vi "Read Item Tag.vi"(8 "error in (no error)":errorcluster, 11 "MenuSelectionMsg in":refnum<class "MenuSelectionMsg.lvclass">) -> (0 "error out":errorcluster, 2 "Item Tag":string, 3 "MenuSelectionMsg out":refnum<class "MenuSelectionMsg.lvclass">)   [LabVIEW 2017, in "ActorEvents.lvlib" / "MenuSelectionMsg.lvclass"]
uses:
  <vilib>/gpm_packages/@cs/mva-viewable/Source/ActorEvents/IEventAggregator Messages/MenuSelectionMsg/MenuSelectionMsg.lvclass
  <vilib>/gpm_packages/@cs/mva-viewable/Source/ActorEvents/IEventAggregator Messages/MenuSelectionMsg/MenuSelectionMsg.lvclass/MenuSelectionMsg.ctl
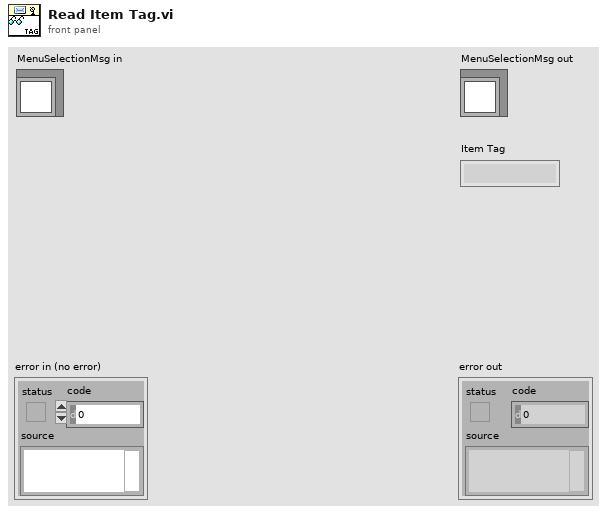
[diagram p1: front panel]
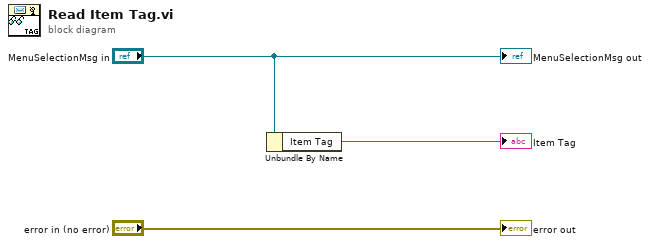
[diagram p0: block diagram]
diagram:
  n1 = Unbundle By Name("MenuSelectionMsg in") -> ("Item Tag"=→"Item Tag":string)
  "error out" <- "error in (no error)"
  "MenuSelectionMsg out" <- "MenuSelectionMsg in"
